vi "OPC DA client write.vi"() -> ()   [LabVIEW 2023]
panel:
  in  "Tab Control":enum32{"Options", "Control"}(tab)=enum."Control"
  in  "OPC Tag":string="opc://localhost/Matrikon.OPC.Simulation.1/Bucket Brigade.Real4"
  in  "Select different OPC Tag":bool
  in  "Temp reading mode":bool
  in  "Manual temperature":dbl=22.0
  in  "Record data":bool
  out "Temperature Chart":dbl(graph)
  out "Temperature":dbl format="%#_4g"
  in  "stop":bool
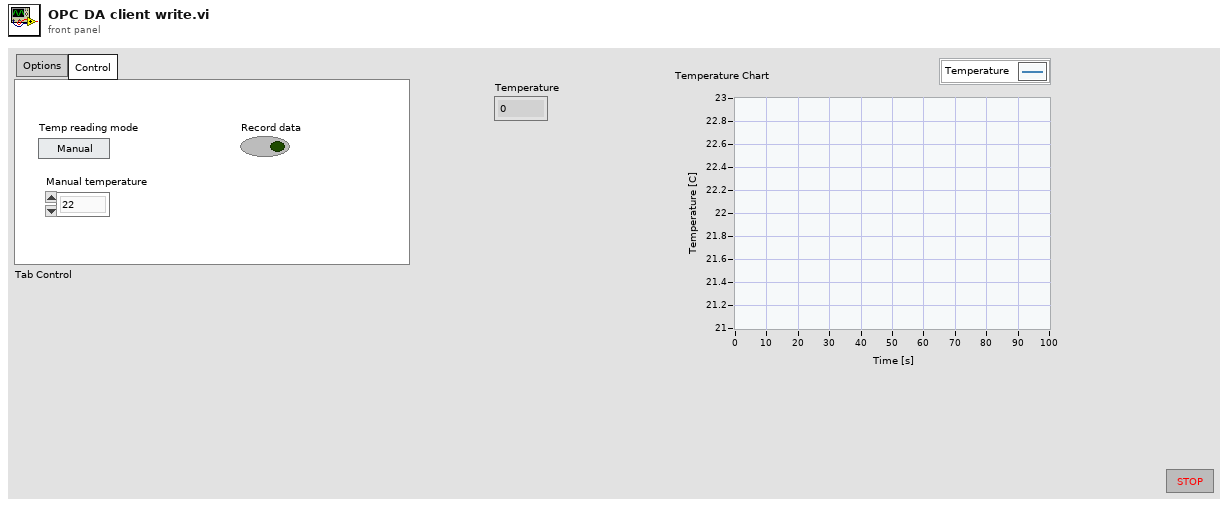
[diagram p1: front panel]
types:
  T1 = enum16{"Read", "Write", "ReadWrite", "BufferedRead", "BufferedReadWrite"}
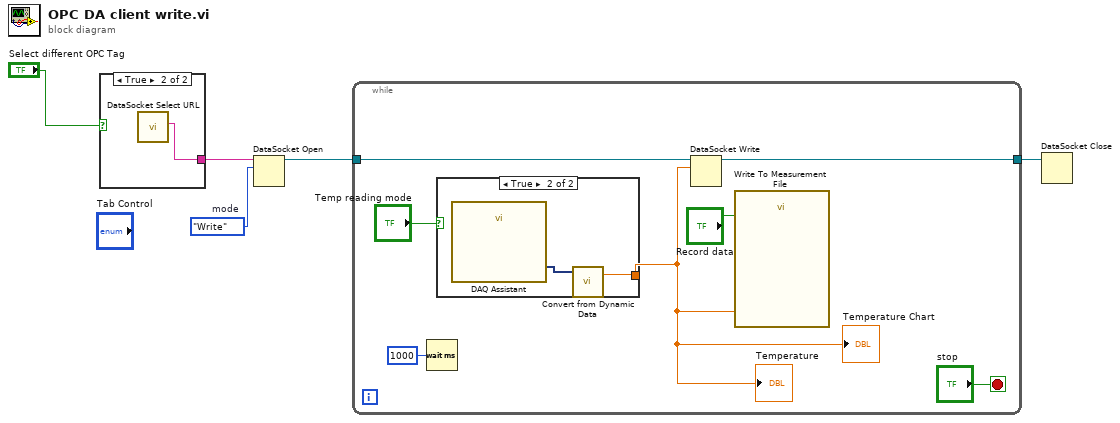
[diagram p0: block diagram]
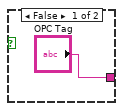
[diagram p2: hidden frame]
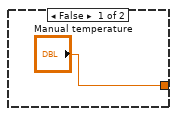
[diagram p3: hidden frame]
diagram:
  w5 = T1."Write"  # mode
  n1 = case shown="True" "Select different OPC Tag" {
    tunnel: ["OPC Tag" w7] -> w2
    frame False {
    }
    frame True {
      n2 = call <vilib>:"DataSocket Select URL.vi"() -> ("URL"=w7:string)  [unwired: 9 in, 2 out]
    }
  }
  n3 = DataSocket Open(10:w5, 11:w2) -> (3:w4:refnum<k13>)  [unwired: 2 in, 1 out]
  n4 = while {
    tunnel: w4 -> [w14]
    tunnel: [w13] -> w3
    stop <- "stop" stop-if-true
    n5 = Wait (ms)(milliseconds to wait=u32 1000) -> ()  [unwired: 1 out]
    n6 = case shown="True" "Temp reading mode" {
      tunnel: ["Manual temperature" w16] -> w8
      frame False {
      }
      frame True {
        n7 = call "DAQ Assistant"() -> ("data"=w17:dynamicdata)  [unwired: 17 in, 2 out]
        n8 = call "Convert from Dynamic Data"("Dynamic Data Type"=w17) -> ("Scalar"=w16:dbl)  [unwired: 3 in]
      }
    }
    "Temperature" <- w8
    "Temperature Chart" <- w8
    n9 = DataSocket Write(10:w8, 11:w14) -> (3:w13:refnum<k13>)  [unwired: 2 in, 2 out]
    n10 = call "Write To Measurement File"("Signals"=w8, "Enable"="Record data") -> ()  [unwired: 15 in, 3 out]
  }
  n11 = DataSocket Close(11:w3) -> ()  [unwired: 2 in, 2 out]
